vi "ORS_WW-RampInt32.vi"(3 "number of sampels from array":dbl[](array[numeric]), 4 "number of samples":i32) -> (1 "output":i32[](array[numeric]))   [LabVIEW 2014]
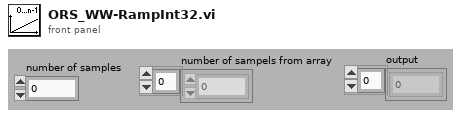
[diagram p1: front panel]
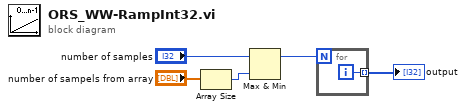
[diagram p0: block diagram]
diagram:
  n1 = Array Size(array="number of sampels from array") -> (size(s)=w2:i32)
  n2 = Max & Min(x="number of samples", y=w2) -> (max(x,y)=w1:i32)  [unwired: 1 out]
  n3 = for {
    N: w1 -> [_]
    tunnel: [w6] -> w5 mode=indexing
    i -> [w6]
  }
  "output" <- w5
